vi "matrix_to_image.vi"(1 "ptb":u8[][](array[numeric])=array241x960[231360 elements]) -> (0 "Image 7":T1(plugin-control))   [LabVIEW 2014]
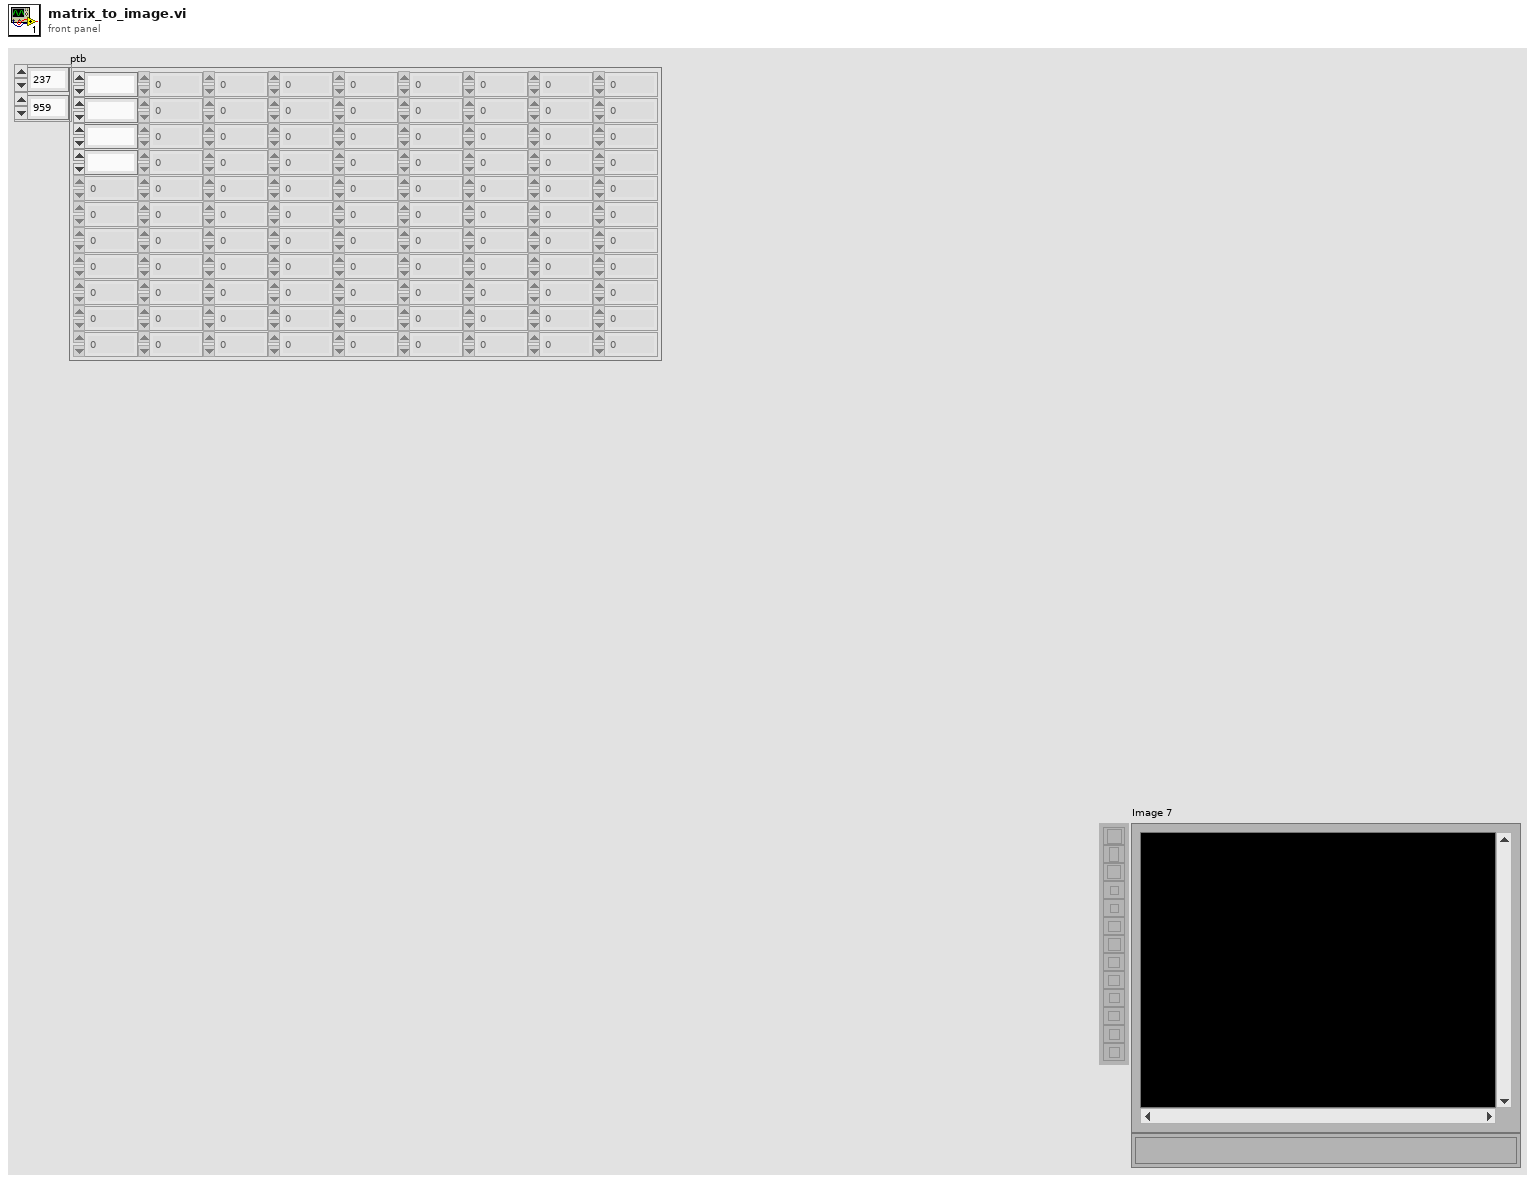
[diagram p1: front panel]
types:
  T1 = typedef "IMAQ Image.ctl" = refnum<image>
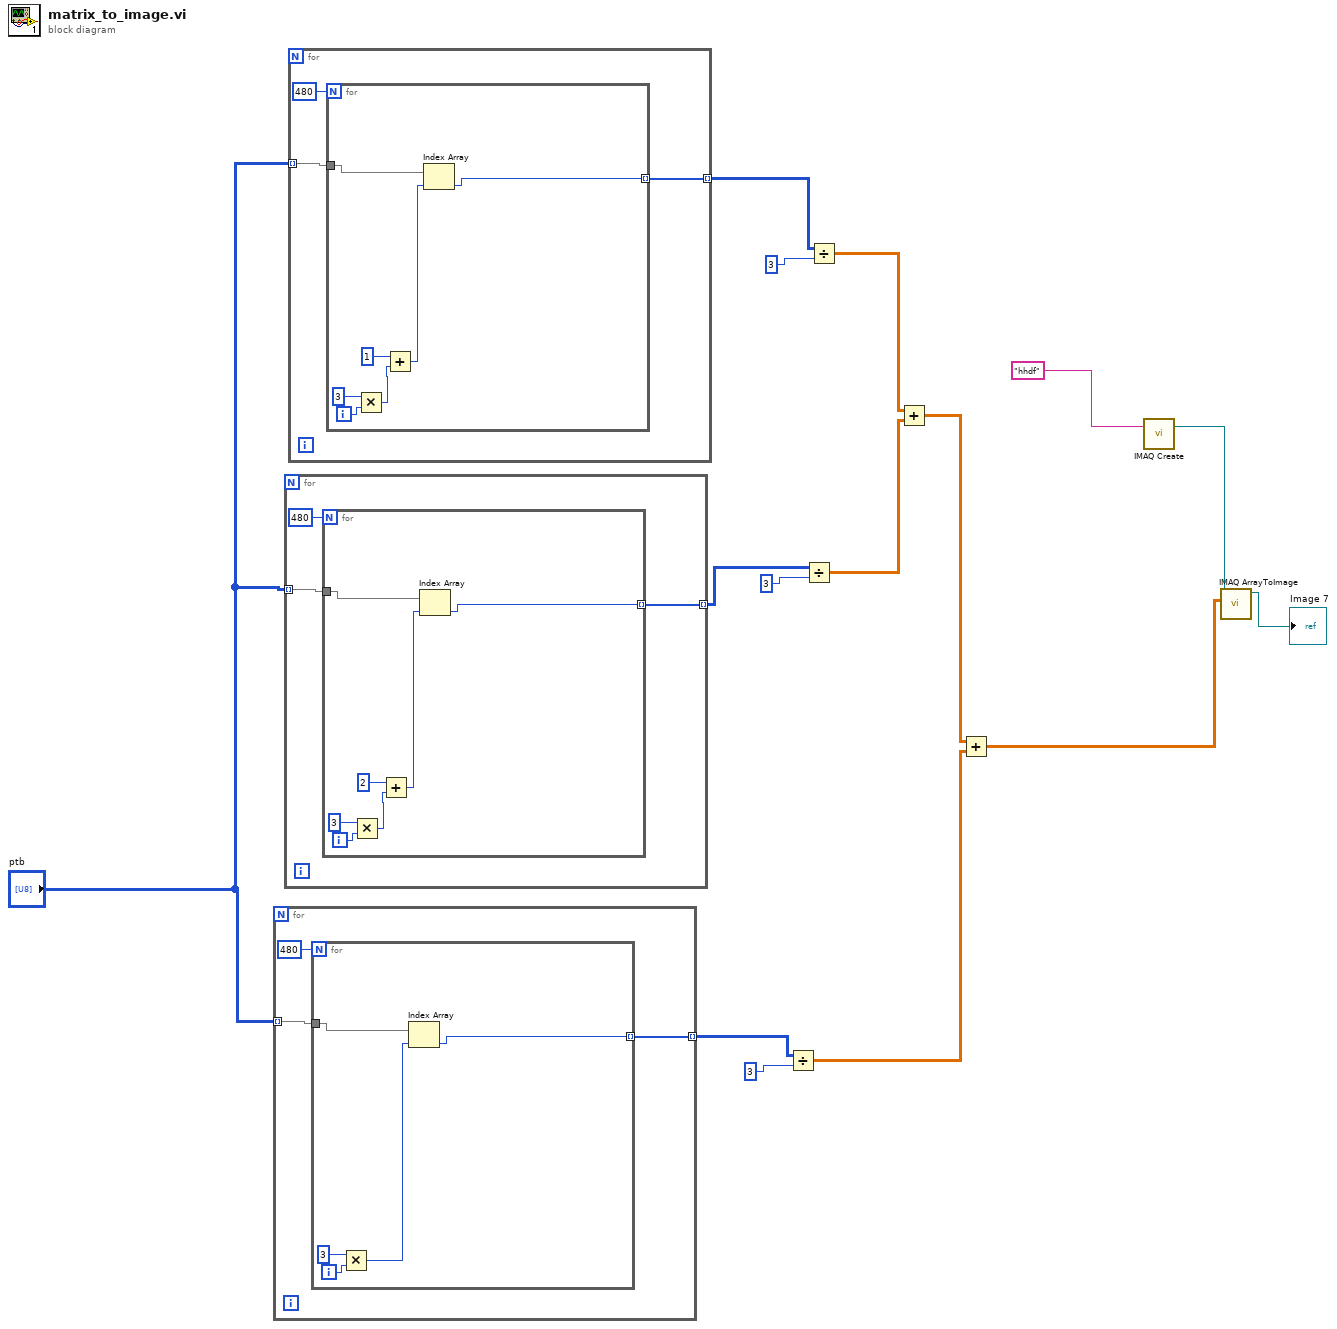
[diagram p0: block diagram]
diagram:
  n1 = for {
    tunnel: "ptb" -> [w18] mode=indexing
    tunnel: [w17] -> w7 mode=indexing
    n2 = for {
      N: 480 -> [_]
      tunnel: w18 -> [w23]
      tunnel: [w19] -> w17 mode=indexing
      i -> [w22]
      n3 = Multiply(x=3, y=w22) -> (x*y=w20:i32)
      n4 = Index Array(array=w23, index=w20) -> (element=w19:u8)
    }
  }
  n5 = for {
    tunnel: "ptb" -> [w26] mode=indexing
    tunnel: [w25] -> w6 mode=indexing
    n6 = for {
      N: 480 -> [_]
      tunnel: w26 -> [w33]
      tunnel: [w30] -> w25 mode=indexing
      i -> [w32]
      n7 = Multiply(x=3, y=w32) -> (x*y=w29:i32)
      n8 = Add(x=2, y=w29) -> (x+y=w27:i32)
      n9 = Index Array(array=w33, index=w27) -> (element=w30:u8)
    }
  }
  n10 = for {
    tunnel: "ptb" -> [w36] mode=indexing
    tunnel: [w35] -> w11 mode=indexing
    n11 = for {
      N: 480 -> [_]
      tunnel: w36 -> [w43]
      tunnel: [w40] -> w35 mode=indexing
      i -> [w42]
      n12 = Multiply(x=3, y=w42) -> (x*y=w39:i32)
      n13 = Add(x=1, y=w39) -> (x+y=w37:i32)
      n14 = Index Array(array=w43, index=w37) -> (element=w40:u8)
    }
  }
  n15 = Divide(x=w7, y=3) -> (x/y=w2:dbl[][])
  n16 = Divide(x=w6, y=3) -> (x/y=w4:dbl[][])
  n17 = Divide(x=w11, y=3) -> (x/y=w5:dbl[][])
  n18 = Add(x=w5, y=w4) -> (x+y=w3:dbl[][])
  n19 = Add(x=w3, y=w2) -> (x+y=w1:dbl[][])
  n20 = call "IMAQ Create"("Image Name"="hhdf") -> ("New Image"=w13:T1)  [unwired: 4 in, 1 out]
  n21 = call "IMAQ ArrayToImage"("Image Pixels (U8)"=w1, "Image"=w13) -> ("Image Out"=→"Image 7":T1)  [unwired: 8 in, 1 out]
